vi "event_setup_stop.vi"(7 "NewVal":bool, 8 "error in (no error)":errorcluster, 9 "reference cluster in":T1, 11 "Boolean in":refnum<vi>) -> (0 "error out":errorcluster)   [LabVIEW 2016]
uses:
  Type Definitions/reference_cluster.ctl
  Type Definitions/vars_settings.ctl
  Type Definitions/stim_type.ctl
  Type Definitions/vars_runtime.ctl
  Type Definitions/data.ctl
  Type Definitions/notifier_elements_GUI.ctl
  Type Definitions/notifier_elements_DAQ.ctl
  Type Definitions/notifier_elements_write.ctl
  Type Definitions/control_references.ctl
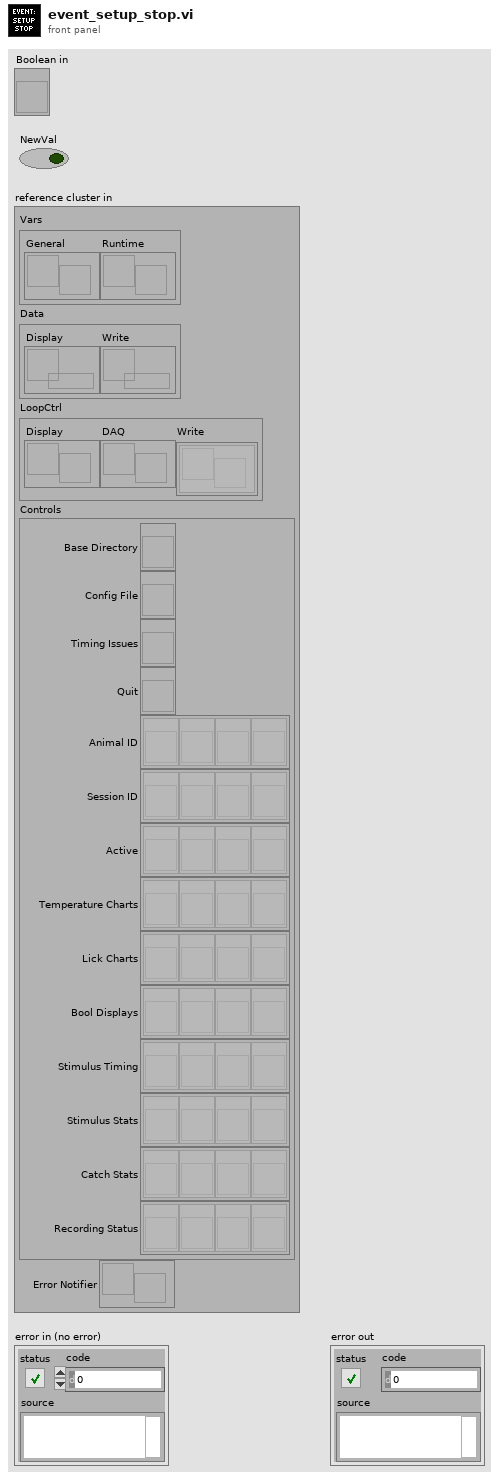
[diagram p1: front panel]
types:
  T1 = typedef "reference_cluster.ctl" = cluster{"Vars":cluster{"General":refnum<notifier>, "Runtime":refnum<notifier>}, "Data":cluster{"Display":refnum<queue>, "Write":refnum<queue>}, "LoopCtrl":cluster{"Display":refnum<notifier>, "DAQ":refnum<notifier>, "Write":refnum<notifier>[]}, "Controls":T2, "Error Notifier":refnum<notifier>}
  T2 = typedef "control_references.ctl" = cluster{"Base Directory":refnum<vi>, "Config File":refnum<vi>, "Timing Issues":refnum<vi>, "Quit":refnum<vi>, "Animal ID":refnum<vi>[], "Session ID":refnum<vi>[], "Active":refnum<vi>[], "Temperature Charts":refnum<vi>[], "Lick Charts":refnum<vi>[], "Bool Displays":refnum<vi>[], "Stimulus Timing":refnum<vi>[], "Stimulus Stats":refnum<vi>[], "Catch Stats":refnum<vi>[], "Recording Status":refnum<vi>[]}
  T3 = enum8{"Enabled", "Disabled", "Disabled and Grayed Out"}
  T4 = typedef "notifier_elements_write.ctl" = enum16{"Initialize", "Pause", "Write Data", "Close Files", "Quit"}
  T5 = enum8{"Enabled", "Disabled", "Disabled and Grayed Out"}[]
  T6 = typedef "vars_settings.ctl" = cluster{"base directory":path, "data directory":path, "active":bool, "running":bool, "pairing":bool, "clean tubes":bool, "animal ID":u16, "session ID":u16, "base temp":dbl, "d wait min":u16, "d wait max":u16, "d timeout":u16, "d reward":u16, "idx stim":u16, "timeout win":u16, "lick win":i32[], "stim type":T7[], "stim amps":dbl[], "d stim":u16[], "d ramp":u16[], "f vibration":u16[], "f squarewave":u8[], "stim shape":dbl[][], "catch":u8[]}
  T7 = typedef "stim_type.ctl" = enum16{"pulse", "vibration", "square", "sine"}
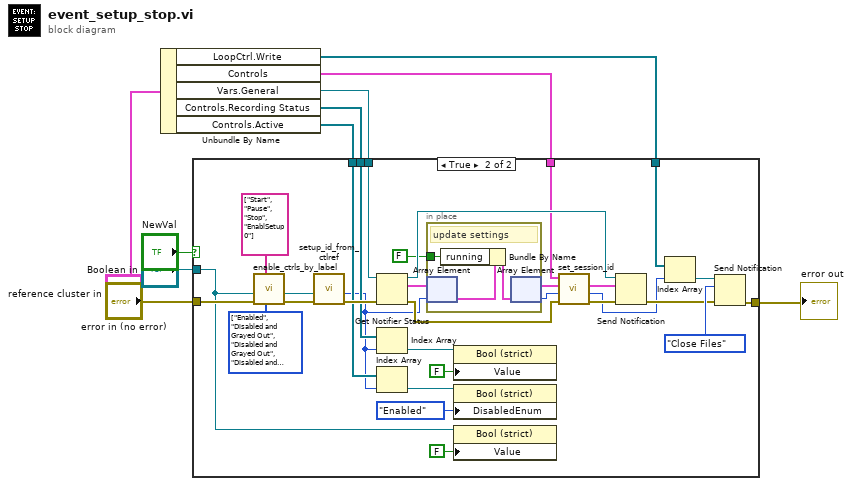
[diagram p0: block diagram]
diagram:
  n1 = Unbundle By Name("reference cluster in") -> ("LoopCtrl.Write"=w4:refnum<notifier>[], "Controls"=w8:T2, "Vars.General"=w7:refnum<notifier>, "Controls.Recording Status"=w9:refnum<vi>[], "Controls.Active"=w10:refnum<vi>[])
  n2 = case shown="True" "NewVal" {
    tunnel: [w11 w31] -> w1
    tunnel: "Boolean in" -> [_ w13]
    tunnel: "error in (no error)" -> [w11 w39]
    tunnel: w4 -> [_ w42]
    tunnel: w7 -> [_ w32]
    tunnel: w8 -> [_ w28]
    tunnel: w9 -> [_ w21]
    tunnel: w10 -> [_ w19]
    frame False {
    }
    frame True {
      w38 = T5 [enum."Enabled", enum."Disabled and Grayed Out", enum."Disabled and Grayed Out", enum."Disabled and Grayed Out"] items=["Enabled", "Disabled", "Disabled and Grayed Out"] ("State")
      n3 = call "enable_ctrls_by_label.vi"("States"=w38, "Names"=string[] ["Start", "Pause", "Stop", "EnablSetup 0"], "error in"=w39, "Refnum in"=w13) -> ("error out"=w15:errorcluster, "Refnum out"=w14:refnum<vi>)  [unwired: 6 in]
      n4 = call "setup_id_from_ctlref.vi"("error in"=w15, "Ctl Refnum"=w14) -> ("error out"=w33:errorcluster, "setup ID"=w18:u16)  [unwired: 6 in]
      n5 = Get Notifier Status(notifier=w32, error in (no error)=w33) -> (notifier out=w37:refnum<notifier>, current notification=w36:T6[], error out=w30:errorcluster)  [unwired: 2 out]
      n6 = Index Array(array=w21, index=w18) -> (element=w23:refnum<vi>)
      n7 = Index Array(array=w19, index=w18) -> (element=w20:refnum<vi>)
      n8 = in-place {
        in-place-border: FALSE ("NewVal") -> [w44]
        # "update settings"
        n9 = in-place-array #1(w36, w18) -> (w45:T6)
        n10 = Bundle By Name(cluster=w45, "running"=w44) -> (w43:T6)
        n11 = in-place-array #1(w43) -> (w27:T6[], w26:i32)
      }
      n12 = property class="Bool (strict)"(reference=w23, "Value"=FALSE) -> ()  [unwired: 1 in, 2 out]
      n13 = property class="Bool (strict)"(reference=w20, "DisabledEnum"=T3."Enabled" ("Disabled")) -> ()  [unwired: 1 in, 2 out]
      n14 = property class="Bool (strict)"(reference=w13, "Value"=FALSE) -> ()  [unwired: 1 in, 2 out]
      n15 = call "set_session_id.vi"("control cluster in"=w28, "settings in"=w27, "setup ID"=w26, "error in"=w30) -> ("settings out"=w24:T6[], "Setup ID"=w25:i32, "error out"=w29:errorcluster)  [unwired: 3 in, 1 out]
      n16 = Send Notification(notification=w24, notifier=w37, error in (no error)=w29) -> (error out=w35:errorcluster)  [unwired: 1 out]
      n17 = Index Array(array=w42, index=w25) -> (element=w41:refnum<notifier>)
      n18 = Send Notification(notification=notifier_elements_write."Close Files", notifier=w41, error in (no error)=w35) -> (error out=w31:errorcluster)  [unwired: 1 out]
    }
  }
  "error out" <- w1
